vi "v3.1.vi"() -> ()   [LabVIEW 2018]
uses:
  <vilib>/DAQmx/read.llb/DAQmx Read (Analog 1D DBL NChan 1Samp).vi
  <extravilib>/ChannelInstances/High Speed Stream-c(a[.](c(dbl,dbl,dbl,dbl)),stamp,a[.](dbl),c(dbl,dbl,dbl,dbl,dbl,dbl,dbl))/_Read For Replicate.vi
  <extravilib>/ChannelInstances/High Speed Stream-c(a[.](c(dbl,dbl,dbl,dbl)),stamp,a[.](dbl),c(dbl,dbl,dbl,dbl,dbl,dbl,dbl))/Instantiate.vi
  <extravilib>/ChannelInstances/High Speed Stream-c(a[.](c(dbl,dbl,dbl,dbl)),stamp,a[.](dbl),c(dbl,dbl,dbl,dbl,dbl,dbl,dbl))/)Channel.vi
  <extravilib>/ChannelInstances/High Speed Stream-c(a[.](c(dbl,dbl,dbl,dbl)),stamp,a[.](dbl),c(dbl,dbl,dbl,dbl,dbl,dbl,dbl))/Abort Signal/Init Signal.vi
  <vilib>/Utility/file.llb/Write Delimited Spreadsheet (string).vi
  <vilib>/DAQmx/create/channels.llb/DAQmx Create Channel (AI-Temperature-Thermocouple).vi
  <vilib>/DAQmx/configure/timing.llb/DAQmx Timing (Sample Clock).vi
  <vilib>/DAQmx/miscellaneous.llb/DAQmx Fill In Error Info.vi
  <extravilib>/ChannelInstances/High Speed Stream-c(a[.](c(dbl,dbl,dbl,dbl)),stamp,a[.](dbl),c(dbl,dbl,dbl,dbl,dbl,dbl,dbl)).lvlib
panel:
  out "x-y":dbl
  out "UI Current Time":timestamp format="%<%X\n%x>T"
  out "Rig Temperatures":T1
  out "DAQ Current Time":timestamp format="%<%X\n%x>T"
  in  "file path (dialog if empty)":path
  out "Enum":T2(ring)
  in  "Start Recording?":bool
  in  "Stop Recording?":bool
  in  "Flowrate Control":dbl
  out "Status":T3(ring)
  in  "OK Button":bool
  in  "DAQ Properties":cluster{"Sample Rate [Hz]":dbl}={"Sample Rate [Hz]"=1.0} {"Sample Rate [Hz]" min=0.1 max=10000.0 step=1.0}
  # "Rig Temperatures [ °C]"
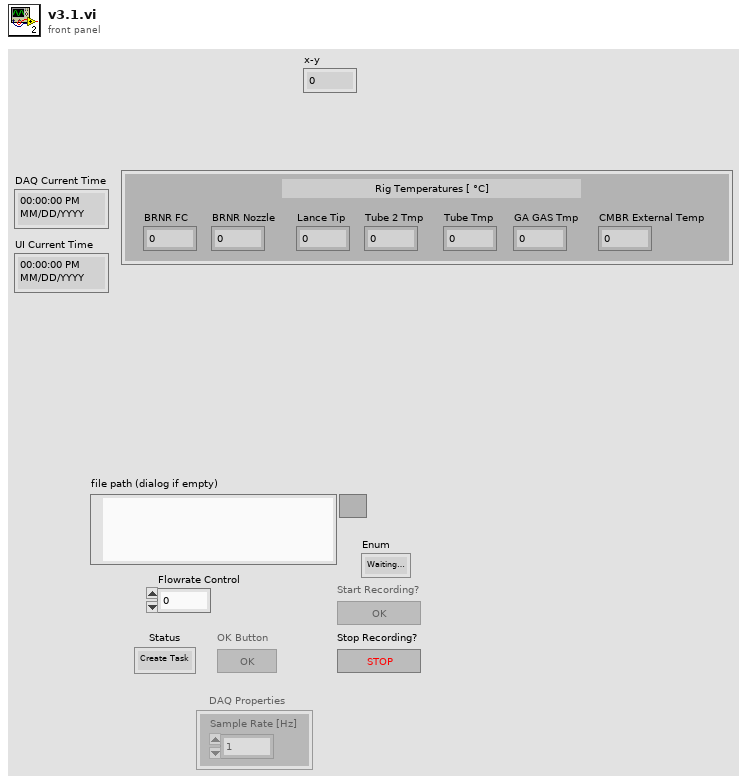
[diagram p1: front panel]
types:
  T1 = cluster{"BRNR FC":dbl, "BRNR Nozzle":dbl, "Lance Tip":dbl, "Tube 2 Tmp":dbl, "Tube Tmp":dbl, "GA GAS Tmp":dbl, "CMBR External Temp":dbl}
  T2 = enum16{"Waiting to record", "Creating Spreadsheet", "Recording", "Finished Recording"}
  T3 = enum16{"Create Task", "Change Settings", "Check Settings", "Read Data", "End Task"}
  T4 = enum8{"Enabled", "Disabled", "Disabled and Grayed Out"}
  T5 = cluster{"Flowrate Data":cluster{"Line Number":dbl, "Temperature":dbl, "Pressure":dbl, "Flowrate":dbl}[], "Current Time":timestamp, "DAQmx Data":dbl[], "Rig Temperatures":cluster{"BRNR FC":dbl, "BRNR Nozzle":dbl, "Lance Tip":dbl, "Tube 2 Tmp":dbl, "Tube Tmp":dbl, "GA GAS Tmp":dbl, "Chamber External Temp":dbl}}
  T6 = cluster{"Line Number":dbl, "Temperature":dbl, "Pressure":dbl, "Flowrate":dbl}[]
  T7 = cluster{"BRNR FC":dbl, "BRNR Nozzle":dbl, "Lance Tip":dbl, "Tube 2 Tmp":dbl, "Tube Tmp":dbl, "GA GAS Tmp":dbl, "Chamber External Temp":dbl}
  T8 = typedef "High Speed Stream-c(a[.](c(dbl,dbl,dbl,dbl)),stamp,a[.](dbl),c(dbl,dbl,dbl,dbl,dbl,dbl,dbl)).lvlib/)Channel.ctl" = refnum<queue>
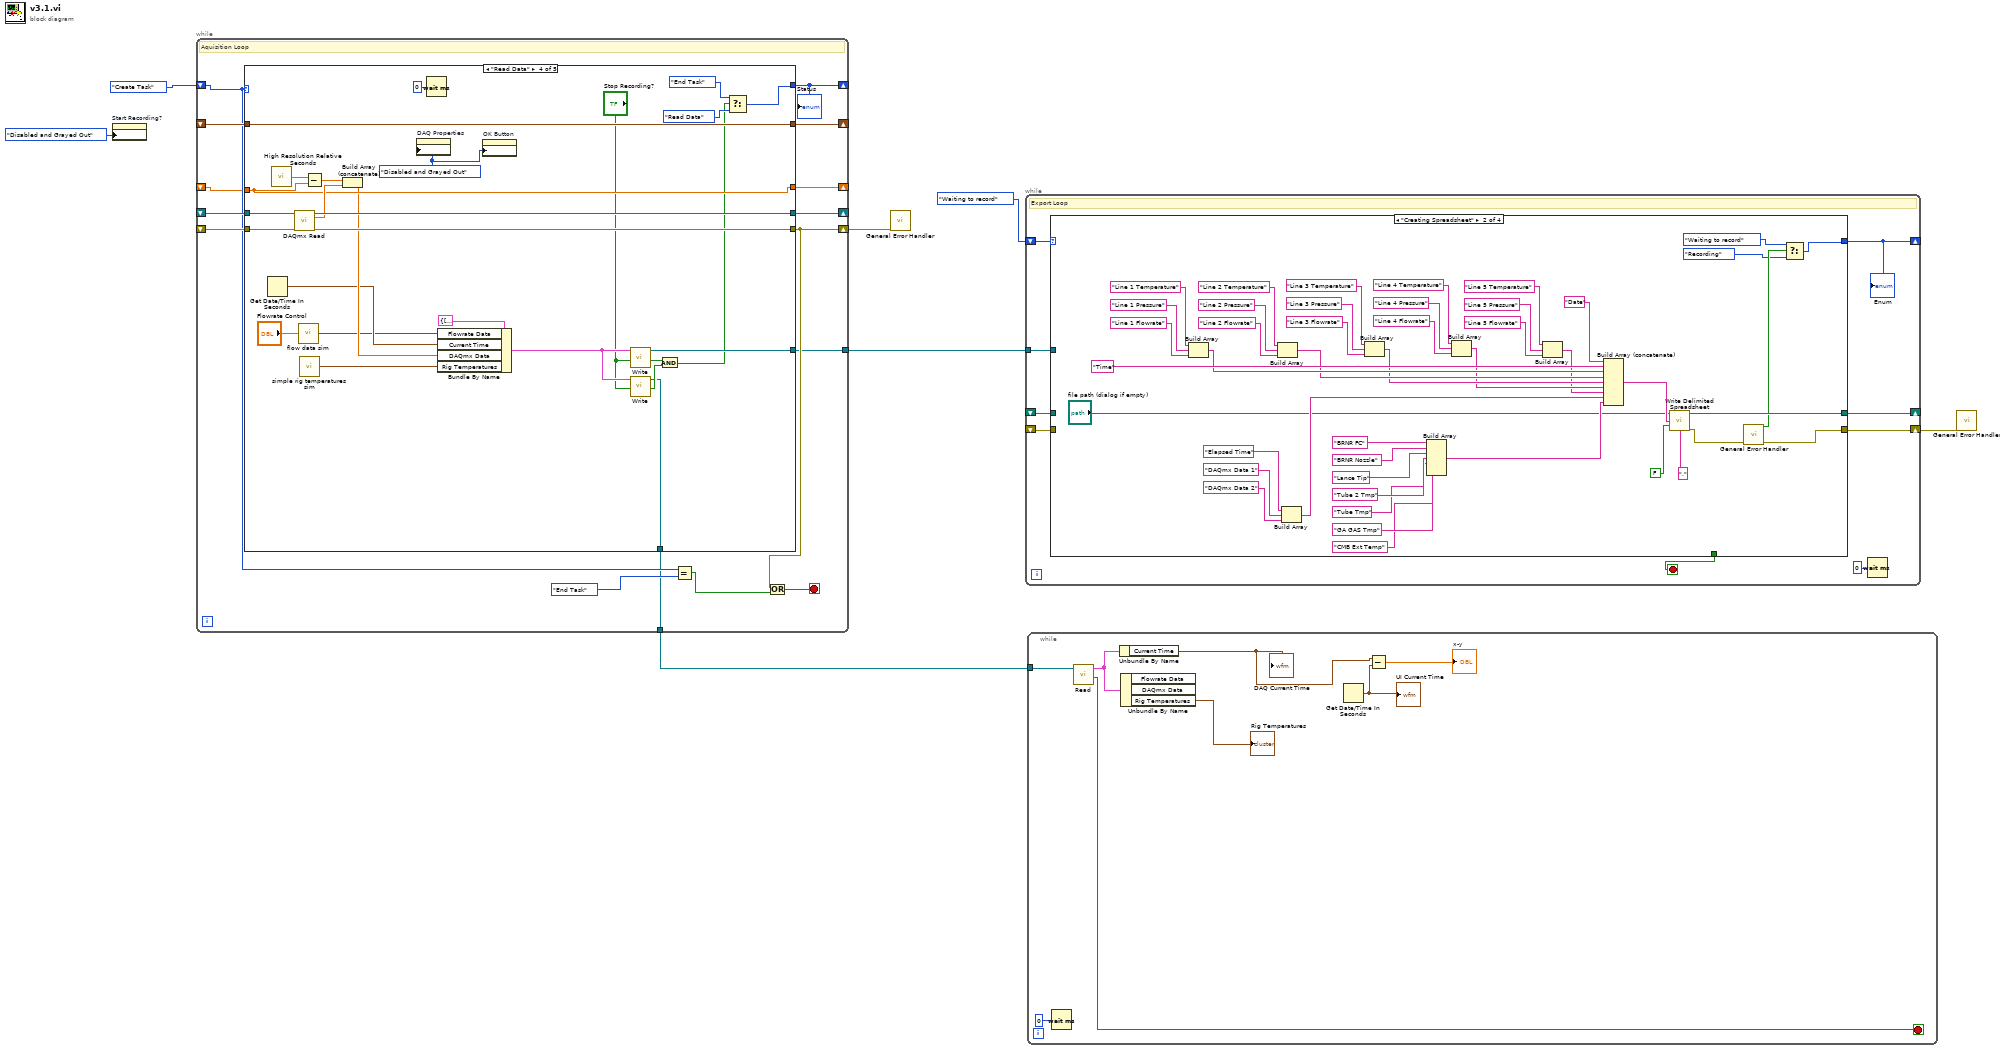
[diagram p0: block diagram]
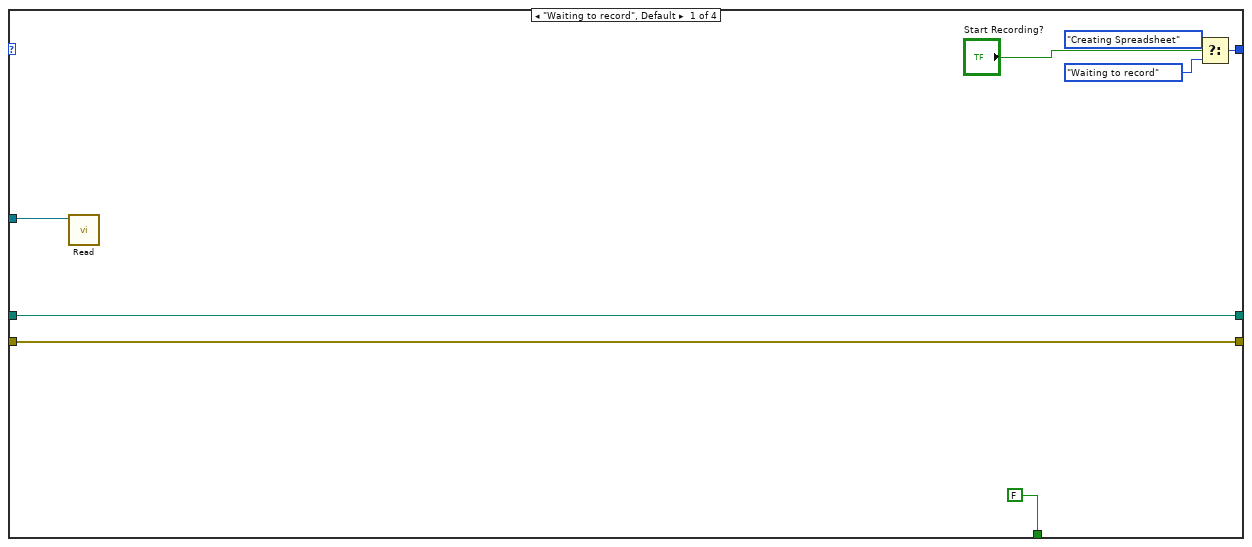
[diagram p2: hidden frame]
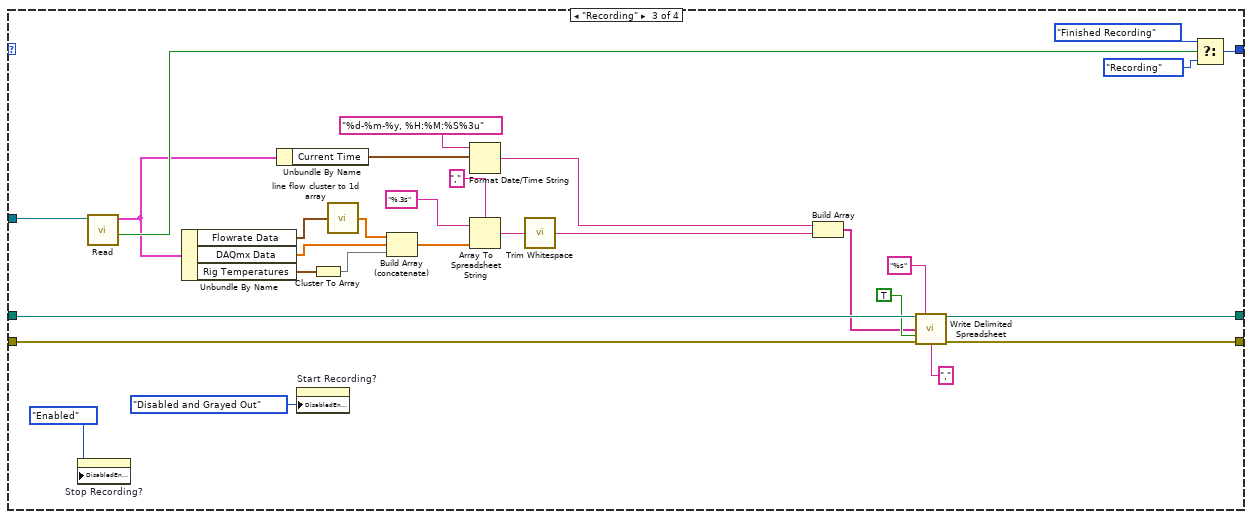
[diagram p3: hidden frame]
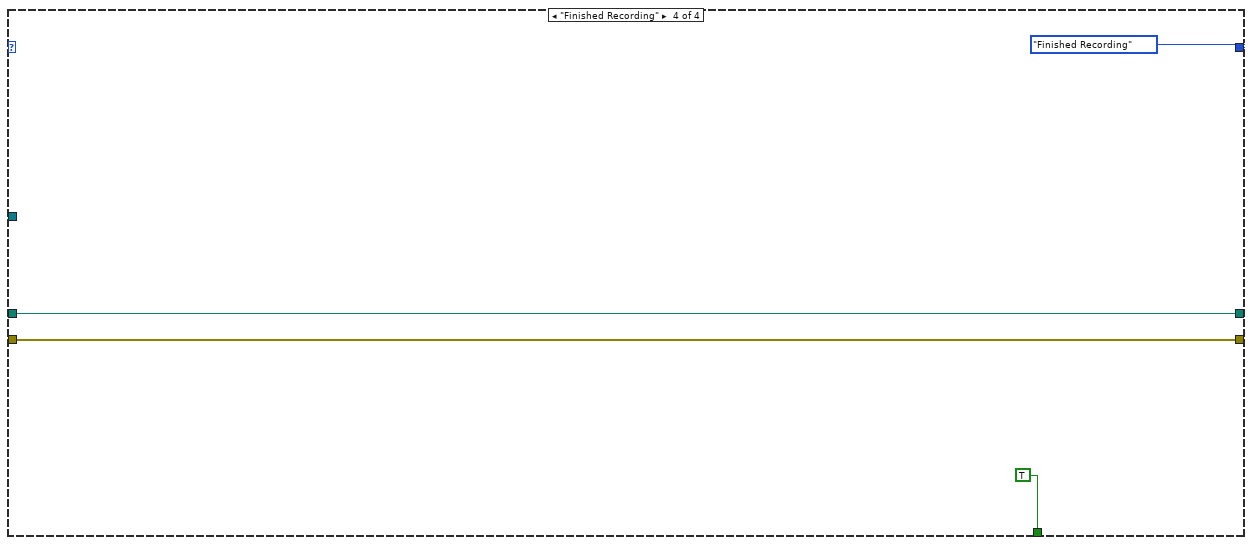
[diagram p4: hidden frame]
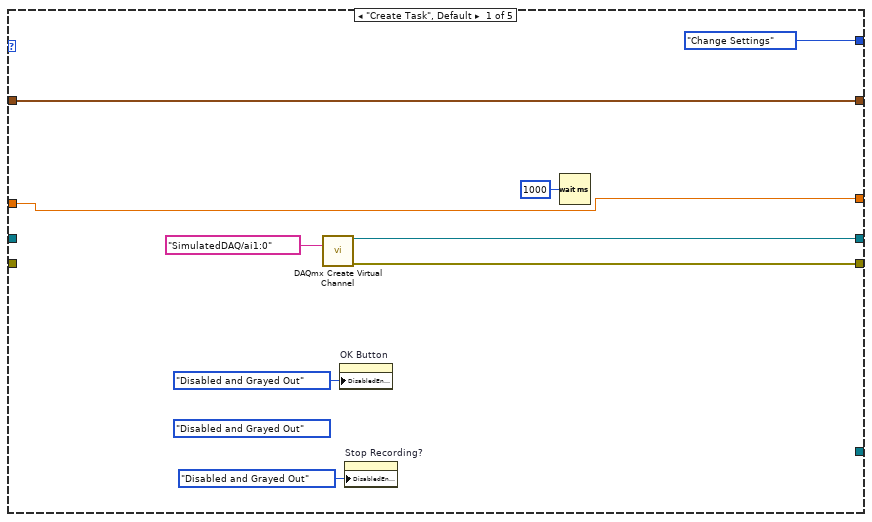
[diagram p5: hidden frame]
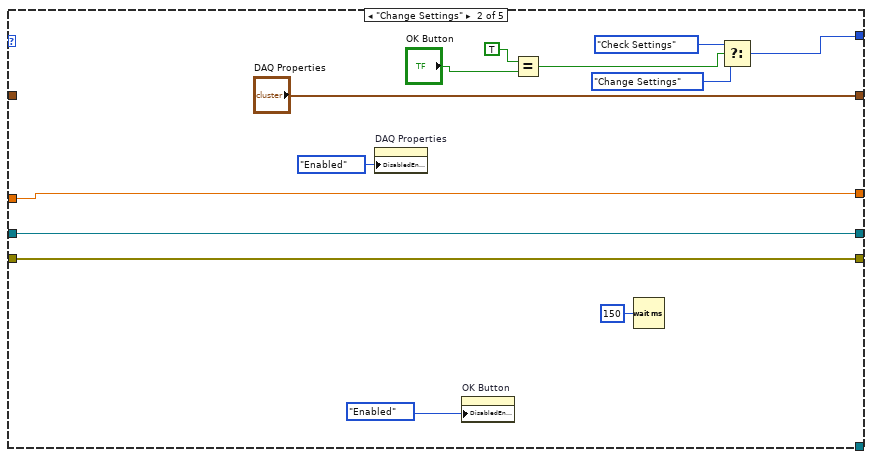
[diagram p6: hidden frame]
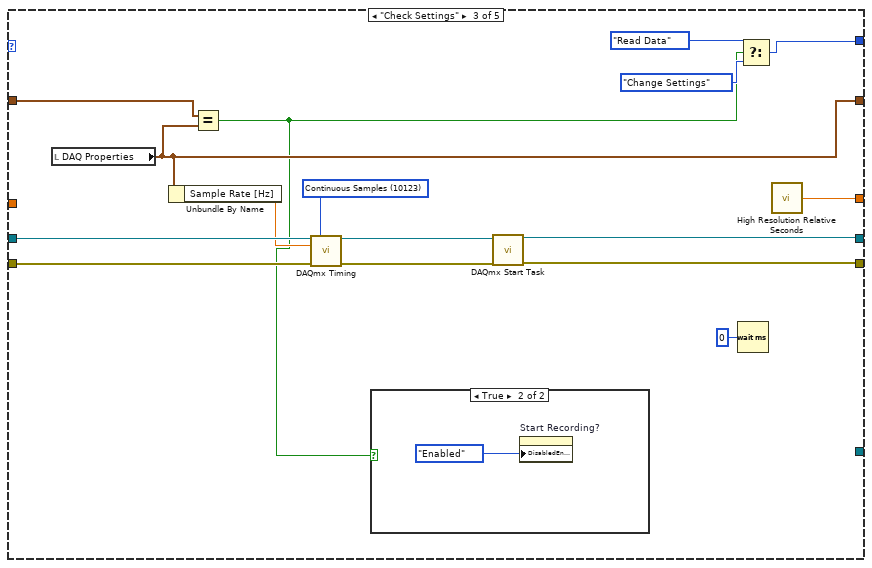
[diagram p7: hidden frame]
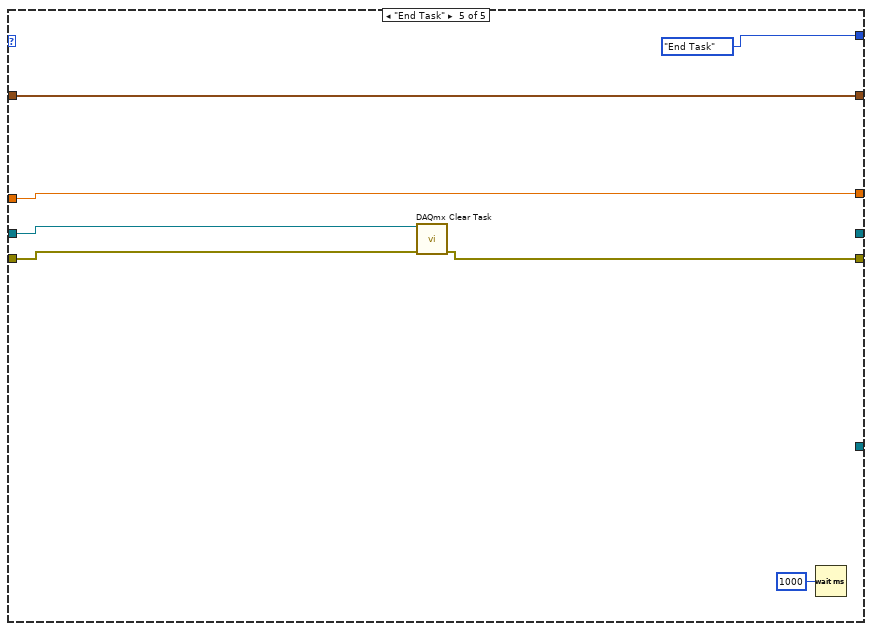
[diagram p9: hidden frame]
diagram:
  n1 = property on="Start Recording?" class="Bool"("DisabledEnum"=T4."Disabled and Grayed Out" ("Disabled")) -> ()  [unwired: 2 in, 2 out]
  n2 = while {
    shift-right: [w17] -> _
    shift-left: T3."Create Task" -> [w13]
    shift-right: [w22] -> _
    shift-left: _ -> [w20]
    shift-right: [w16] -> w3
    shift-left: _ -> [w19]
    shift-right: [w21] -> _
    shift-left: _ -> [w18]
    shift-right: [w12] -> _
    shift-left: _ -> [w11]
    tunnel: [w9] -> w5
    tunnel: [w8] -> w1
    stop <- w10 stop-if-true
    # "Aquisition Loop"
    n3 = case shown="\"Read Data\"" w13 {
      tunnel: [w31 w44 w49 w85 _] -> w22
      tunnel: [w30 w43 w48 w84 w95] -> w16
      tunnel: [T3."Change Settings" w37 w56 w82 T3."End Task"] -> w17
      tunnel: [w27 "DAQ Properties" w52 w86 w94] -> w21
      tunnel: w20 -> [_ w44 w55 w88 w92]
      tunnel: w19 -> [_ w43 w54 w87 w91]
      tunnel: w18 -> [w27 _ w60 w86 w94]
      tunnel: [w25 w34 w46 w76 w90] -> w12
      tunnel: w11 -> [w25 w34 _ w76 w90]
      tunnel: [_ _ _ w69 _] -> w9
      tunnel: [_ _ _ w62 _] -> w8
      frame "Create Task", Default {
        (unwired) T4."Disabled and Grayed Out" ("Disabled")
        n4 = call-poly <vilib>:"DAQmx Create Virtual Channel.vi"("physical channels"=tag "SimulatedDAQ/ai1:0") -> ("task out"=w31:refnum<k21>, "error out"=w30:errorcluster)  [unwired: 13 in]
        n5 = property on="OK Button" class="Bool"("DisabledEnum"=T4."Disabled and Grayed Out" ("Disabled")) -> ()  [unwired: 2 in, 2 out]
        n6 = property on="Stop Recording?" class="Bool"("DisabledEnum"=T4."Disabled and Grayed Out" ("Disabled")) -> ()  [unwired: 2 in, 2 out]
        n7 = Wait (ms)(milliseconds to wait=u32 1000) -> ()  [unwired: 1 out]
      }
      frame "Change Settings" {
        n8 = property on="DAQ Properties" class="Clust (strict)"("DisabledEnum"=T4."Enabled" ("Disabled")) -> ()  [unwired: 2 in, 2 out]
        n9 = property on="OK Button" class="Bool"("DisabledEnum"=T4."Enabled" ("Disabled")) -> ()  [unwired: 2 in, 2 out]
        n10 = Equal?(x=TRUE, y="OK Button") -> (x = y?=w39:bool)
        n11 = Wait (ms)(milliseconds to wait=u32 150) -> ()  [unwired: 1 out]
        n12 = Select(t=T3."Check Settings", s=w39, f=T3."Change Settings") -> (s? t:f=w37:T3)
      }
      frame "Check Settings" {
        w47 = 10123 items=["Finite Samples"=10178, "Continuous Samples"=10123, "Hardware Timed Single Point"=12522] ("sample mode")
        n13 = local read "DAQ Properties"() -> (w52:cluster{"Sample Rate [Hz]":dbl})
        n14 = Unbundle By Name(w52) -> ("Sample Rate [Hz]"=w53:dbl)
        n15 = Equal?(x=w60, y=w52) -> (x = y?=w45:bool)
        n16 = call-poly <vilib>:"DAQmx Timing.vi"("task/channels in"=w55, "sample mode"=w47, "rate"=w53, "error in"=w54) -> ("task out"=w51:refnum<k21>, "error out"=w50:errorcluster)  [unwired: 10 in]
        n17 = case shown="True" w45 {
          frame False {
          }
          frame True {
            n18 = property on="Start Recording?" class="Bool"("DisabledEnum"=T4."Enabled" ("Disabled")) -> ()  [unwired: 2 in, 2 out]
          }
        }
        n19 = call <vilib>:"DAQmx Start Task.vi"("task/channels in"=w51, "error in"=w50) -> ("task out"=w49:refnum<k21>, "error out"=w48:errorcluster)  [unwired: 12 in]
        n20 = Wait (ms)(milliseconds to wait=u32 0) -> ()  [unwired: 1 out]
        n21 = Select(t=T3."Read Data", s=w45, f=T3."Change Settings") -> (s? t:f=w56:T3)
        n22 = call <vilib>:"High Resolution Relative Seconds.vi"() -> ("relative seconds"=w46:dbl)
      }
      frame "Read Data" {
        w68 = T4."Disabled and Grayed Out" ("Disabled")
        n23 = Get Date/Time In Seconds() -> (seconds since 1Jan1904=w72:timestamp)
        n24 = call <vilib>:"High Resolution Relative Seconds.vi"() -> ("relative seconds"=w79:dbl)
        n25 = call-poly <vilib>:"DAQmx Read.vi"("task/channels in"=w88, "error in"=w87) -> ("task out"=w85:refnum<k21>, "data"=w78:dbl[], "error out"=w84:errorcluster)  [unwired: 11 in]
        n26 = call "flow data sim.vi"("Boondoggle Input"="Flowrate Control") -> ("Flowrate Data"=w71:T6)
        n27 = call "simple rig temperatures sim.vi"() -> ("Rig Temperatures"=w70:T7)
        n28 = Subtract(x=w79, y=w76) -> (x-y=w77:dbl)
        n29 = Build Array (concatenate)(w77, w78) -> (w73:dbl[])
        n30 = property on="DAQ Properties" class="Clust (strict)"("DisabledEnum"=w68) -> ()  [unwired: 2 in, 2 out]
        n31 = Wait (ms)(milliseconds to wait=u32 0) -> ()  [unwired: 1 out]
        n32 = Bundle By Name(cluster=T5 {"Flowrate Data"=[{"Line Number"=1.0, "Temperature"=17.480721541683437, "Pressure"=24.0, "Flowrate"=0.0}, {"Line Number"=2.0, "Temperature"=21.850901927104296, "Pressure"=30.0, "Flowrate"=0.0}, {"Line Number"=3.0, "Temperature"=26.221082312525155, "Pressure"=36.0, "Flowrate"=0.0}, {"Line Number"=4.0, "Temperature"=30.591262697946018, "Pressure"=42.00000000000001, "Flowrate"=0.0}, {"Line Number"=5.0, "Temperature"=34.96144308336687, "Pressure"=48.0, "Flowrate"=0.0}], "Current Time"=timestamp(0 s since 1904-01-01), "DAQmx Data"=[], "Rig Temperatures"={"BRNR FC"=0.0, "BRNR Nozzle"=0.0, "Lance Tip"=0.0, "Tube 2 Tmp"=0.0, "Tube Tmp"=0.0, "GA GAS Tmp"=0.0, "Chamber External Temp"=0.0}}, "Flowrate Data"=w71, "Current Time"=w72, "DAQmx Data"=w73, "Rig Temperatures"=w70) -> (w67:T5)
        n33 = property on="OK Button" class="Bool"("DisabledEnum"=w68) -> ()  [unwired: 2 in, 2 out]
        n34 = call <extravilib>:"Write.vi"("last element? (F)"="Stop Recording?", "element"=w67) -> ("done?"=w65:bool, "channel"=w69:T8)  [unwired: 7 in, 1 out]
        n35 = call <extravilib>:"Write.vi"("last element? (F)"="Stop Recording?", "element"=w67) -> ("done?"=w64:bool, "channel"=w62:T8)  [unwired: 7 in, 1 out]
        n36 = And(x=w65, y=w64) -> (x .and. y?=w63:bool)
        n37 = Select(t=T3."End Task", s=w63, f=T3."Read Data") -> (s? t:f=w82:T3)
      }
      frame "End Task" {
        n38 = call <vilib>:"DAQmx Clear Task.vi"("task in"=w92, "error in"=w91) -> ("error out"=w95:errorcluster)  [unwired: 13 in]
        n39 = Wait (ms)(milliseconds to wait=u32 1000) -> ()  [unwired: 1 out]
      }
    }
    "Status" <- w17
    n40 = Equal?(x=w13, y=T3."End Task") -> (x = y?=w14:bool)
    n41 = Or(x=w16, y=w14) -> (x .or. y?=w10:bool)
  }
  n42 = call <vilib>:"General Error Handler.vi"("error in (no error)"=w3) -> ()  [unwired: 10 in, 5 out]
  n43 = while {
    shift-right: [w103] -> _
    shift-left: T2."Waiting to record" -> [w102]
    tunnel: w5 -> [w100]
    shift-right: [w98] -> _
    shift-left: _ -> [w99]
    shift-right: [w97] -> w4
    shift-left: _ -> [w96]
    stop <- w101 stop-if-true
    # "Export Loop"
    n44 = case shown="\"Creating Spreadsheet\"" w102 {
      tunnel: [w109 w115 w185 T2."Finished Recording"] -> w103
      tunnel: [FALSE _ _ TRUE] -> w101
      tunnel: w100 -> [w105 _ w181 _]
      tunnel: w99 -> [w107 _ w178 w188]
      tunnel: [w107 w137 w179 w188] -> w98
      tunnel: [w106 w117 w158 w187] -> w97
      tunnel: w96 -> [w106 _ w169 w187]
      frame "Waiting to record", Default {
        n45 = call <extravilib>:"Read.vi"("channel"=w105) -> ()  [unwired: 6 in, 5 out]
        n46 = Select(t=T2."Creating Spreadsheet", s="Start Recording?", f=T2."Waiting to record") -> (s? t:f=w109:T2)
      }
      frame "Creating Spreadsheet" {
        n47 = Build Array("Line 1 Temperature", "Line 1 Pressure", "Line 1 Flowrate") -> (w141:string[])
        n48 = Build Array("Line 2 Temperature", "Line 2 Pressure", "Line 2 Flowrate") -> (w140:string[])
        n49 = Build Array("Elapsed Time", "DAQmx Data 1", "DAQmx Data 2") -> (w130:string[])
        n50 = Build Array("Line 3 Temperature", "Line 3 Pressure", "Line 3 Flowrate") -> (w139:string[])
        n51 = Build Array("BRNR FC", "BRNR Nozzle", "Lance Tip", "Tube 2 Tmp", "Tube Tmp", "GA GAS Tmp", "CMB Ext Temp") -> (w122:string[])
        n52 = Build Array("Line 4 Temperature", "Line 4 Pressure", "Line 4 Flowrate") -> (w138:string[])
        n53 = Build Array("Line 5 Temperature", "Line 5 Pressure", "Line 5 Flowrate") -> (w131:string[])
        n54 = Build Array (concatenate)("Date", "Time", w141, w140, w139, w138, w131, w130, w122) -> (w136:string[])
        n55 = call-poly <vilib>:"Write Delimited Spreadsheet.vi"("file path (dialog if empty)"="file path (dialog if empty)", "1D data"=w136, "append to file? (new file:F)"=FALSE, "delimiter (\\t)"="," ("delimiter (\\t)")) -> ("new file path (Not A Path if cancelled)"=w137:path, "error out"=w118:errorcluster)  [unwired: 10 in]
        n56 = call <vilib>:"General Error Handler.vi"("error in (no error)"=w118) -> ("error?"=w116:bool, "error out"=w117:errorcluster)  [unwired: 10 in, 3 out]
        n57 = Select(t=T2."Waiting to record", s=w116, f=T2."Recording") -> (s? t:f=w115:T2)
      }
      frame "Recording" {
        n58 = property on="Stop Recording?" class="Bool"("DisabledEnum"=T4."Enabled" ("Disabled")) -> ()  [unwired: 2 in, 2 out]
        n59 = call <extravilib>:"Read.vi"("channel"=w181) -> ("done?"=w180:bool, "element"=w175:T5)  [unwired: 6 in, 3 out]
        n60 = Unbundle By Name(w175) -> ("Flowrate Data"=w176:T6, "DAQmx Data"=w173:dbl[], "Rig Temperatures"=w182:T7)
        n61 = Unbundle By Name(w175) -> ("Current Time"=w160:timestamp)
        n62 = property on="Start Recording?" class="Bool"("DisabledEnum"=T4."Disabled and Grayed Out" ("Disabled")) -> ()  [unwired: 2 in, 2 out]
        n63 = Cluster To Array(cluster=w182) -> (array=w174:dbl[])
        n64 = call "line flow cluster to 1d array.vi"("Flowrate Data"=w176) -> ("Array"=w172:dbl[])
        n65 = Build Array (concatenate)(w172, w173, w174) -> (w171:dbl[])
        n66 = Format Date/Time String(time format string (%c)="%d-%m-%y, %H:%M:%S%3u", seconds (now)=w160) -> (date/time string=w162:string)  [unwired: 1 in]
        n67 = Array To Spreadsheet String(delimiter (Tab)=",", array=w171, 3:"%.3s" ("format string")) -> (spreadsheet string=w166:string)
        n68 = call <vilib>:"Trim Whitespace.vi"("string"=w166) -> ("trimmed string"=w165:string)  [unwired: 1 in]
        n69 = Build Array(w162, w165) -> (w167:string[])
        n70 = call-poly <vilib>:"Write Delimited Spreadsheet.vi"("file path (dialog if empty)"=w178, "format (%s)"="%s", "1D data"=w167, "append to file? (new file:F)"=TRUE, "error in (no error)"=w169, "delimiter (\\t)"="," ("delimiter (\\t)")) -> ("new file path (Not A Path if cancelled)"=w179:path, "error out"=w158:errorcluster)  [unwired: 8 in]
        n71 = Select(t=T2."Finished Recording", s=w180, f=T2."Recording") -> (s? t:f=w185:T2)
      }
      frame "Finished Recording" {
      }
    }
    "Enum" <- w103
    n72 = Wait (ms)(milliseconds to wait=u32 0) -> ()  [unwired: 1 out]
  }
  n73 = while {
    tunnel: w1 -> [w198]
    stop <- w197 stop-if-true
    n74 = Wait (ms)(milliseconds to wait=u32 0) -> ()  [unwired: 1 out]
    n75 = call <extravilib>:"Read.vi"("channel"=w198) -> ("done?"=w197:bool, "element"=w195:T5)  [unwired: 6 in, 3 out]
    n76 = Unbundle By Name(w195) -> ("Current Time"=w193:timestamp)
    "DAQ Current Time" <- w193
    n77 = Unbundle By Name(w195) -> ("Rig Temperatures"=→"Rig Temperatures":T7)  [unwired: 2 out]
    n78 = Get Date/Time In Seconds() -> (seconds since 1Jan1904=w192:timestamp)
    "UI Current Time" <- w192
    n79 = Subtract(x=w193, y=w192) -> (x-y=→"x-y":dbl)
  }
  n80 = call <vilib>:"General Error Handler.vi"("error in (no error)"=w4) -> ()  [unwired: 10 in, 5 out]
